vi "Calcu_STD Pressure_PC.vi"(6 "Resolution":string[][](array[string]), 7 "STD 단위":string, 8 "Cal STD (-)":string[](array[string]), 10 "Cal STD (+)":string[](array[string]), 11 "Condition":string[][](array[string])) -> (0 "배열":dbl[](array[numeric]), 3 "Data Out":string[][](array[string]), 5 "STD Data":string[][](array[string]))   [LabVIEW 2020]
uses:
  Variables/Global_Cal Info.vi
  <vilib>/express/express arith-compare/Formula/XNode/ExpressFormulaBlockNode.xnode
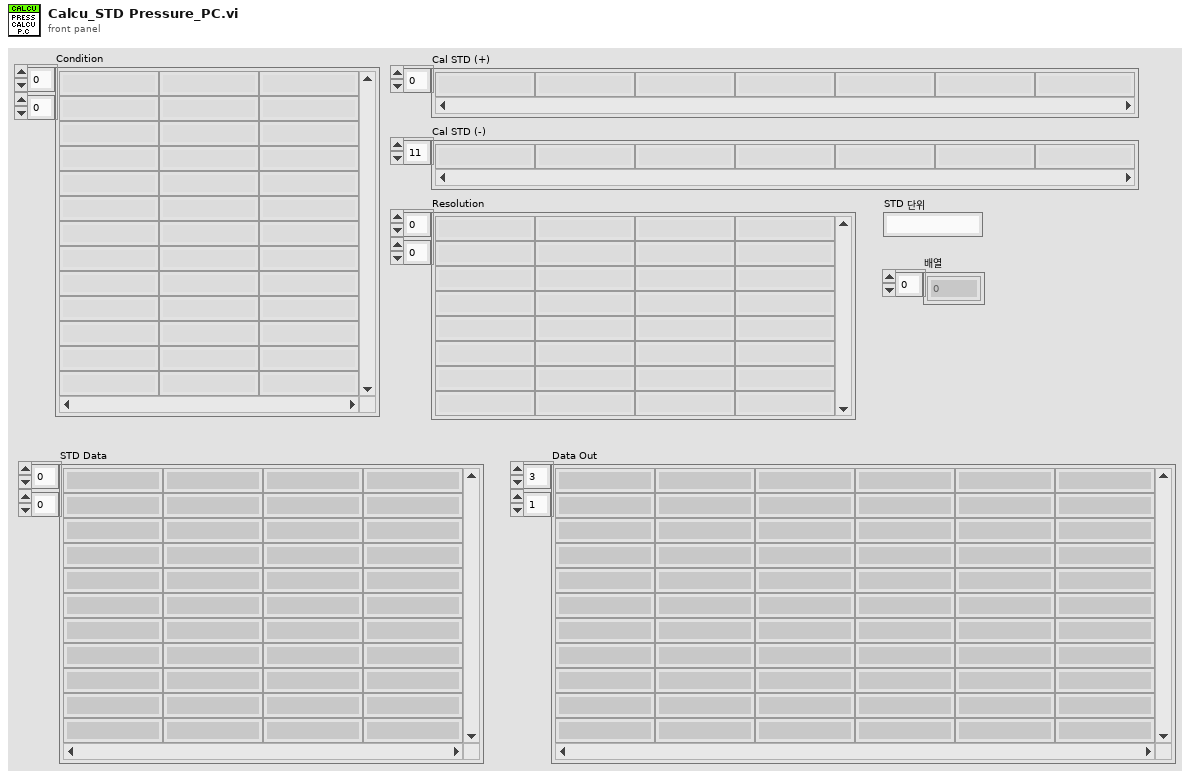
[diagram p1: front panel]
types:
  T1 = cluster{"세부분류코드":string, "형식":string, "옵션":string, "측정기명":string, "EXCEL파일명":string, "TEMP":string}
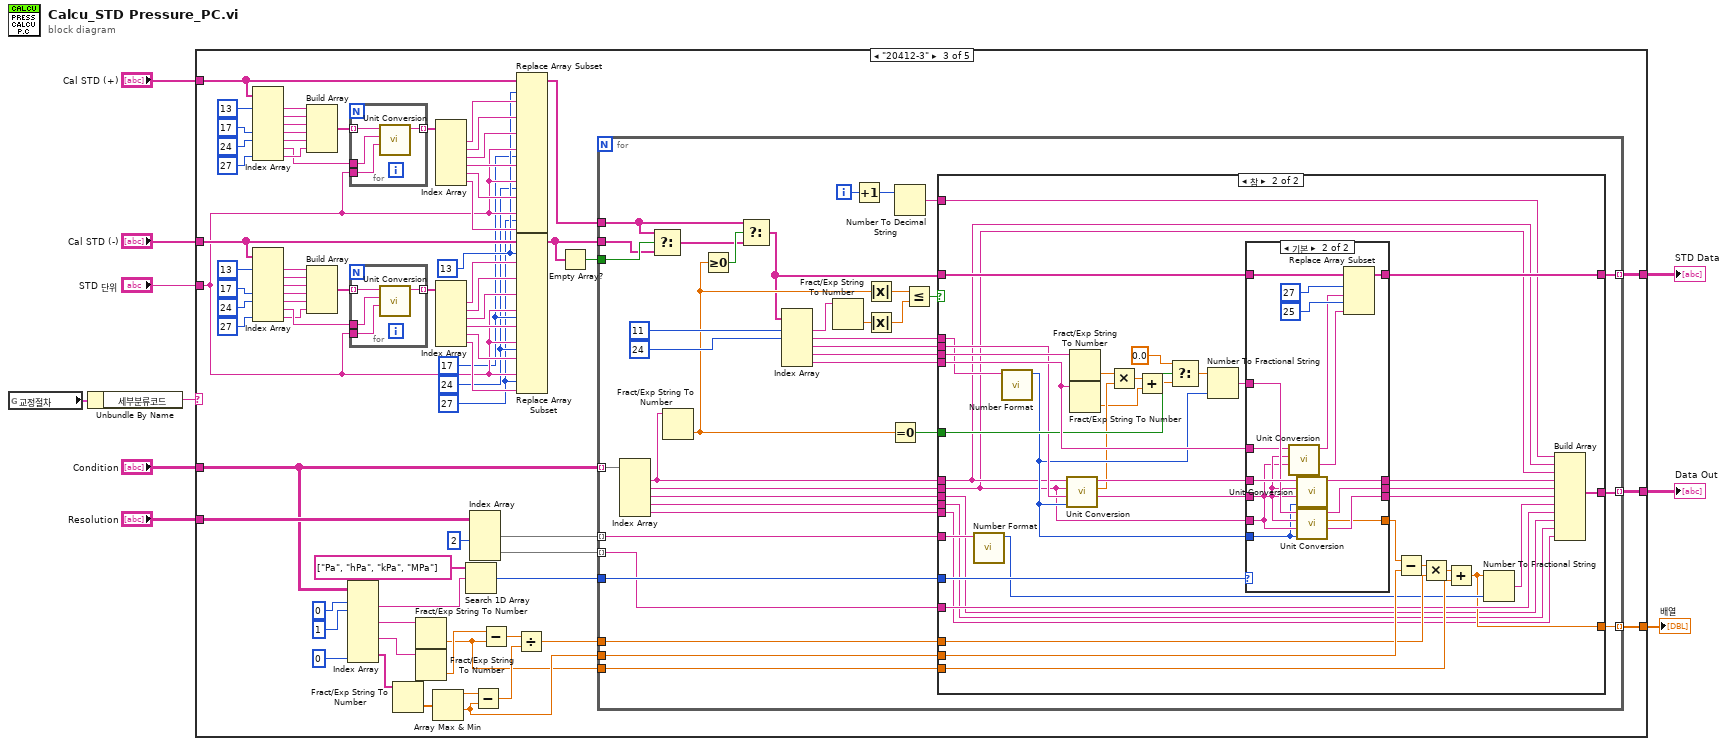
[diagram p0: block diagram]
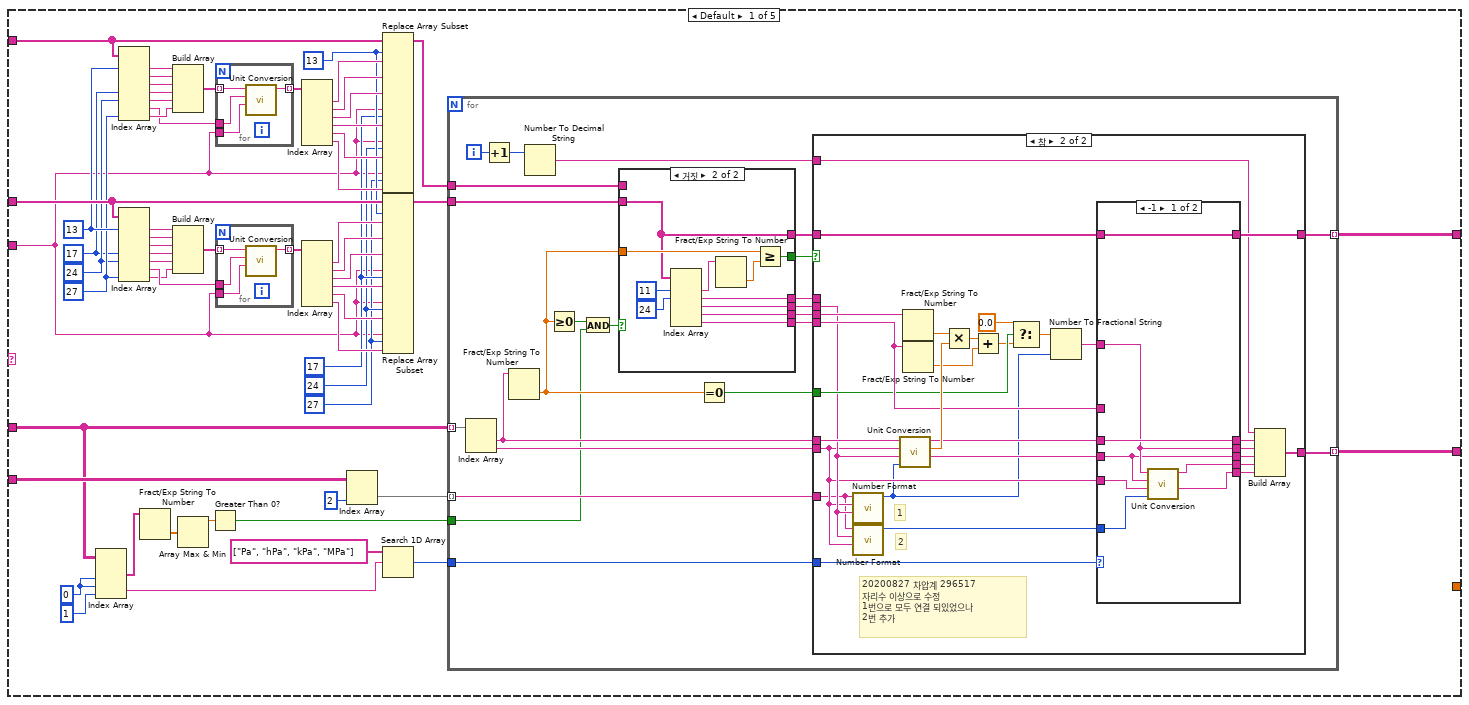
[diagram p2: hidden frame]
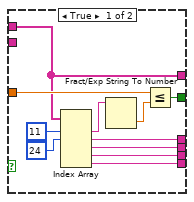
[diagram p3: hidden frame]
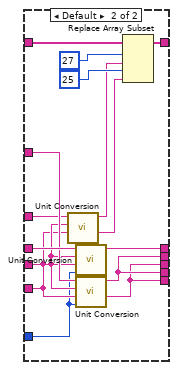
[diagram p5: hidden frame]
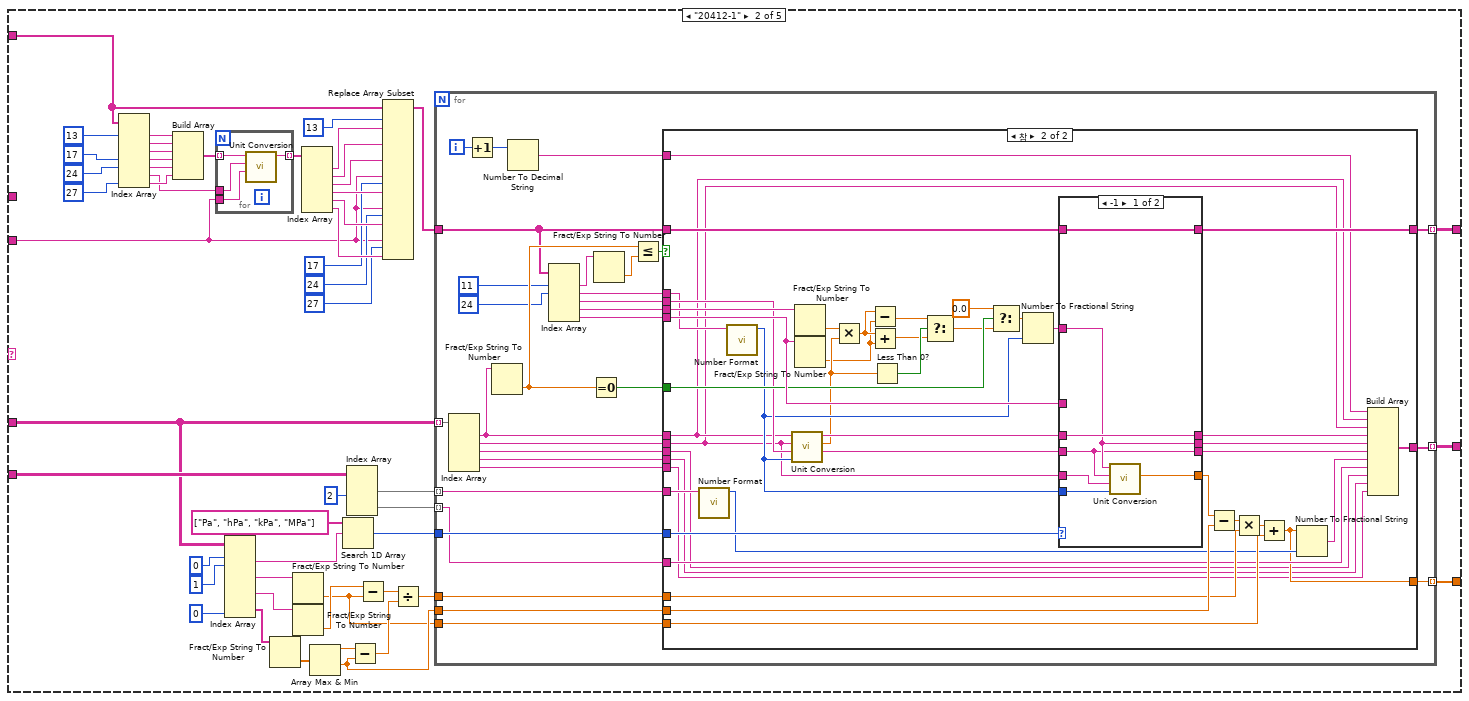
[diagram p6: hidden frame]
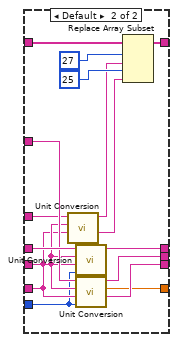
[diagram p8: hidden frame]
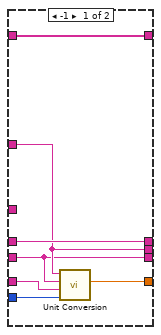
[diagram p10: hidden frame]
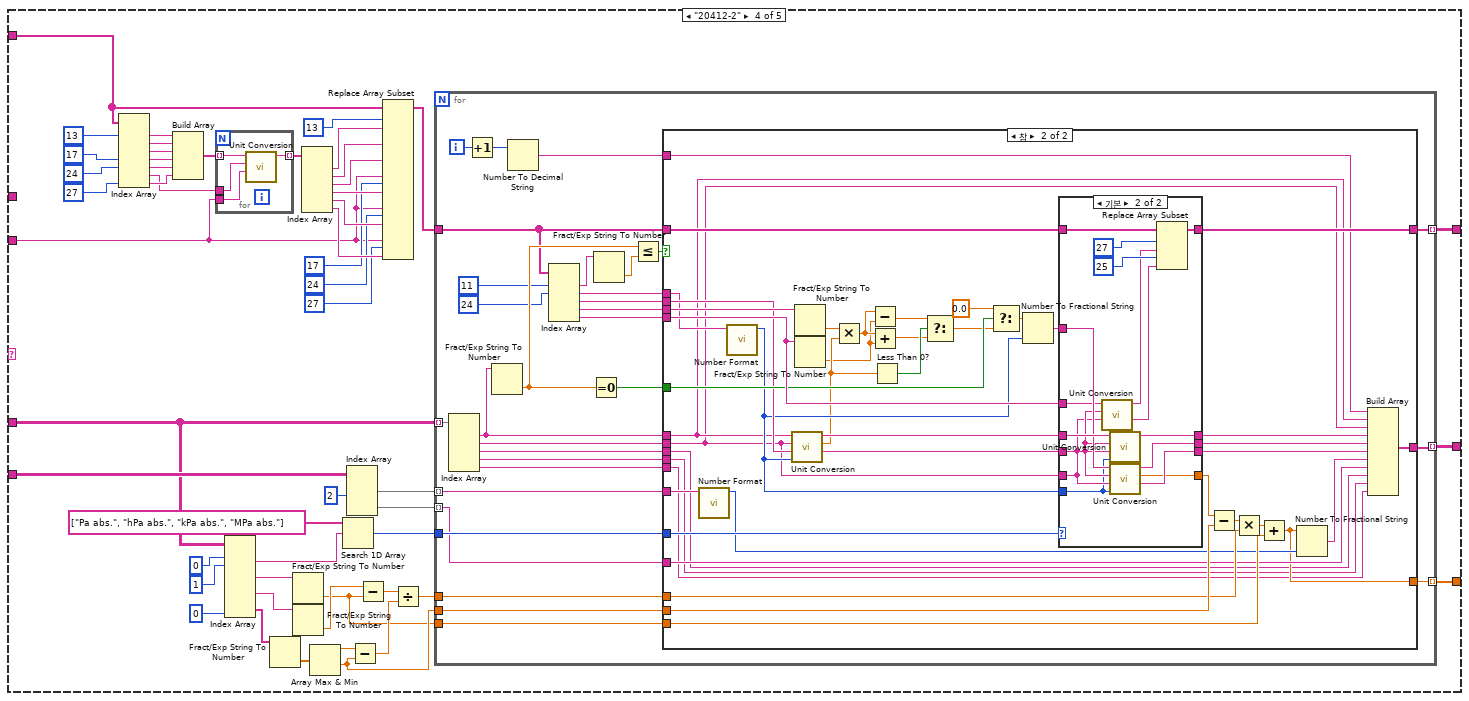
[diagram p11: hidden frame]
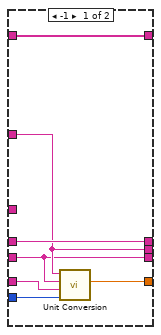
[diagram p13: hidden frame]
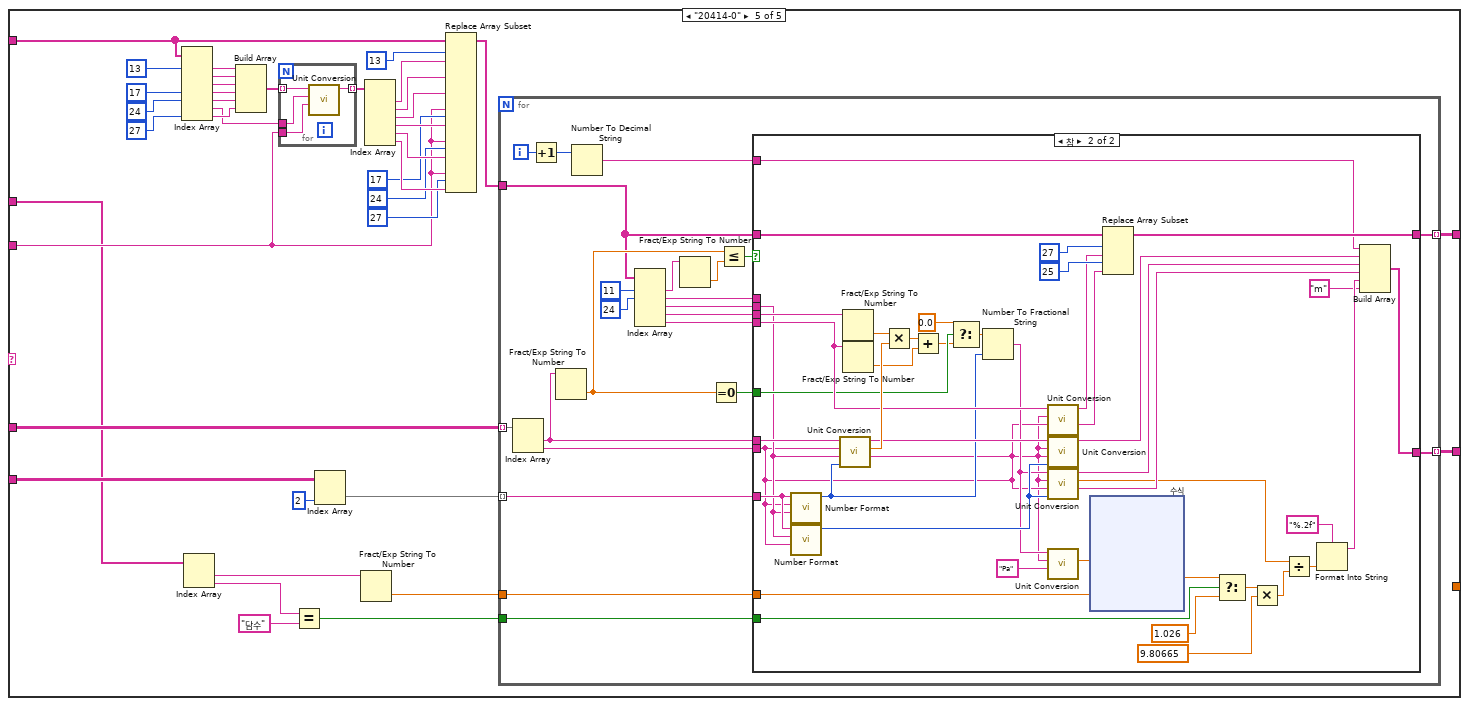
[diagram p14: hidden frame]
diagram:
  n1 = global read "Global_Cal Info.vi" "교정절차"() -> (w3:T1)
  n2 = Unbundle By Name(w3) -> ("세부분류코드"=w2:string)
  n3 = case shown="\"20412-3\"" w2 {
    tunnel: "Resolution" -> [w68 w224 w397 w556 w694]
    tunnel: [w61 w217 w390 w549 w691] -> w9
    tunnel: [w60 w216 w389 w548 w690] -> w8
    tunnel: "Condition" -> [w59 w215 w388 w547 w689]
    tunnel: "Cal STD (+)" -> [w43 w199 w372 w531 w665]
    tunnel: "Cal STD (-)" -> [w26 _ w332 _ w662]
    tunnel: "STD 단위" -> [w16 w189 w331 w521 w664]
    tunnel: [_ w174 w352 w506 _] -> w1
    frame Default {
      w23 = 17 ("인덱스")
      w21 = 27 ("인덱스")
      w22 = 24 ("인덱스")
      w24 = 13 ("인덱스")
      w17 = 17 ("인덱스")
      w19 = 27 ("인덱스")
      w18 = 24 ("인덱스")
      w20 = 13 ("인덱스")
      w11 = 0 ("비활성화된 인덱스 (열)")
      n4 = Index Array(array=w59, index (col) #1=w11, index (row) #2=w11, index (col) #2=1 ("인덱스 (행)")) -> (element #1=w13:string[], element #2=w66:string)  [unwired: 1 in]
      n5 = Index Array(array=w43, index #1=w20, index #4=w17, index #5=w18, index #7=w19) -> (element #1=w58:string, element #2=w57:string, element #3=w56:string, element #4=w54:string, element #5=w53:string, element #6=w52:string, element #7=w55:string)  [unwired: 3 in]
      n6 = Index Array(array=w26, index #1=w20, index #4=w17, index #5=w18, index #7=w19) -> (element #1=w27:string, element #2=w28:string, element #3=w29:string, element #4=w31:string, element #5=w32:string, element #6=w33:string, element #7=w30:string)  [unwired: 3 in]
      n7 = Fract/Exp String To Number(string=w13) -> (number=w14:dbl[])  [unwired: 3 in, 1 out]
      n8 = Build Array(w58, w57, w56, w54, w53, w55) -> (w51:string[])
      n9 = Build Array(w27, w28, w29, w31, w32, w30) -> (w34:string[])
      n10 = Array Max & Min(array=w14) -> (max value=w15:dbl)  [unwired: 3 out]
      n11 = Greater Than 0?(x=w15) -> (x > 0?=w12:bool)
      n12 = for {
        tunnel: w52 -> [w76]
        tunnel: w51 -> [w75] mode=indexing
        tunnel: w16 -> [w74]
        tunnel: [w73] -> w50 mode=indexing
        n13 = call "Unit Conversion.vi"("환산단위"=w74, "입력단위"=w76, "입력값"=w75) -> ("환산값 (string)"=w73:string)  [unwired: 3 in, 5 out]
      }
      n14 = for {
        tunnel: w33 -> [w72]
        tunnel: w34 -> [w71] mode=indexing
        tunnel: w16 -> [w70]
        tunnel: [w69] -> w35 mode=indexing
        n15 = call "Unit Conversion.vi"("환산단위"=w70, "입력단위"=w72, "입력값"=w71) -> ("환산값 (string)"=w69:string)  [unwired: 3 in, 5 out]
      }
      n16 = Index Array(array=w50) -> (element #1=w49:string, element #2=w48:string, element #3=w47:string, element #4=w46:string, element #5=w45:string, element #6=w44:string)  [unwired: 6 in]
      n17 = Index Array(array=w35) -> (element #1=w36:string, element #2=w37:string, element #3=w38:string, element #4=w39:string, element #5=w40:string, element #6=w41:string)  [unwired: 6 in]
      n18 = Index Array(array=w68, index (col)=2 ("비활성화된 인덱스 (열)")) -> (element=w62:string[])  [unwired: 1 in]
      n19 = Replace Array Subset(array=w43, new element #1=w49, index #1=w24, new element #2=w48, new element #3=w47, new element #4=w16, new element #5=w46, index #5=w23, new element #6=w16, new element #7=w45, index #7=w22, new element #8=w16, new element #9=w44, index #9=w21) -> (w42:string[])  [unwired: 5 in]
      n20 = Replace Array Subset(array=w26, new element #1=w36, index #1=w24, new element #2=w37, new element #3=w38, new element #4=w16, new element #5=w39, index #5=w23, new element #6=w16, new element #7=w40, index #7=w22, new element #8=w16, new element #9=w41, index #9=w21) -> (w25:string[])  [unwired: 5 in]
      n21 = Search 1D Array(1D array=string[] ["Pa", "hPa", "kPa", "MPa"], element=w66) -> (index of element=w67:i32)  [unwired: 1 in]
      n22 = for {
        tunnel: w59 -> [w99] mode=indexing
        tunnel: [w97] -> w60 mode=indexing
        tunnel: w42 -> [w98]
        tunnel: [w96] -> w61 mode=indexing
        tunnel: w62 -> [w92] mode=indexing
        tunnel: w67 -> [w93]
        tunnel: w25 -> [w88]
        tunnel: w12 -> [w77]
        i -> [w91]
        n23 = Index Array(array=w99) -> (element #1=w94:string, element #2=w95:string)  [unwired: 2 in]
        n24 = Increment(x=w91) -> (x+1=w90:i32)
        n25 = Fract/Exp String To Number(string=w94) -> (number=w87:dbl)  [unwired: 3 in, 1 out]
        n26 = Number To Decimal String(number=w90) -> (decimal integer string=w89:string)  [unwired: 1 in]
        n27 = Greater Or Equal To 0?(x=w87) -> (x >= 0?=w79:bool)
        n28 = And(x=w79, y=w77) -> (x .and. y?=w78:bool)
        n29 = case shown="거짓" w78 {
          tunnel: w98 -> [w100 _]
          tunnel: [w110 w121] -> w86
          tunnel: [w109 w120] -> w85
          tunnel: [w108 w119] -> w84
          tunnel: [w107 w118] -> w83
          tunnel: w87 -> [w106 w117]
          tunnel: [w101 w112] -> w82
          tunnel: w88 -> [_ w111]
          tunnel: [w100 w111] -> w81
          frame True {
            n30 = Index Array(array=w100, index #1=11 ("인덱스"), index #2=24 ("인덱스")) -> (element #1=w103:string, element #2=w101:string, element #3=w108:string, element #4=w107:string, element #5=w109:string)  [unwired: 3 in]
            n31 = Fract/Exp String To Number(string=w103) -> (number=w105:dbl)  [unwired: 3 in, 1 out]
            n32 = Less Or Equal?(x=w106, y=w105) -> (x <= y?=w110:bool)
          }
          frame False {
            n33 = Index Array(array=w111, index #1=11 ("인덱스"), index #2=24 ("인덱스")) -> (element #1=w114:string, element #2=w112:string, element #3=w119:string, element #4=w118:string, element #5=w120:string)  [unwired: 3 in]
            n34 = Fract/Exp String To Number(string=w114) -> (number=w116:dbl)  [unwired: 3 in, 1 out]
            n35 = Greater Or Equal?(x=w117, y=w116) -> (x >= y?=w121:bool)
          }
        }
        n36 = Equal To 0?(x=w87) -> (x = 0?=w80:bool)
        n37 = case shown="참" w86 {
          tunnel: [_ w149] -> w96
          tunnel: w89 -> [_ w134]
          tunnel: w81 -> [_ w137]
          tunnel: [_ w136] -> w97
          tunnel: w84 -> [_ w127]
          tunnel: w85 -> [_ w135]
          tunnel: w95 -> [_ w126]
          tunnel: w94 -> [_ w144]
          tunnel: w83 -> [_ w147]
          tunnel: w82 -> [_ _]
          tunnel: w93 -> [_ w143]
          tunnel: w92 -> [_ w122]
          tunnel: w80 -> [_ w133]
          frame False {
          }
          frame True {
            # "2"
            # "1"
            # "20200827 차압계 296517\n자리수 이상으로 수정\n1번으로 모두 연결 되있었으나\n2번 추가"
            n38 = call "Number Format.vi"("기준단위"=w127, "입력단위"=w126, "입력값"=w122) -> ("정밀도(단위적용)"=w123:i32)  [unwired: 8 in]
            n39 = call "Number Format.vi"("기준단위"=w126, "입력단위"=w127, "입력값"=w122) -> ("정밀도(단위적용)"=w124:i32)  [unwired: 8 in]
            n40 = call "Unit Conversion.vi"("소수점 자리수"=w123, "환산단위"=w127, "입력단위"=w126, "입력값"=w144) -> ("환산단위"=w128:string, "환산값 (DBL)"=w148:dbl, "환산값 (string)"=w129:string)  [unwired: 2 in, 3 out]
            n41 = Fract/Exp String To Number(string=w147) -> (number=w146:dbl)  [unwired: 3 in, 1 out]
            n42 = Fract/Exp String To Number(string=w135) -> (number=w145:dbl)  [unwired: 3 in, 1 out]
            n43 = Multiply(x=w146, y=w148) -> (x*y=w150:dbl)
            n44 = Add(x=w150, y=w145) -> (x+y=w132:dbl)
            n45 = Select(t=0.0, s=w133, f=w132) -> (s? t:f=w130:dbl)
            n46 = Number To Fractional String(number=w130, precision (6)=w123) -> (F-format string=w125:string)  [unwired: 2 in]
            n47 = case shown="-1" w143 {
              tunnel: w129 -> [w158 w173]
              tunnel: w126 -> [w151 w160]
              tunnel: w125 -> [w155 w172]
              tunnel: [w158 w171] -> w142
              tunnel: [w155 w170] -> w141
              tunnel: [w152 w169] -> w140
              tunnel: [w157 w170] -> w139
              tunnel: [w156 w169] -> w138
              tunnel: w124 -> [w154 w159]
              tunnel: w128 -> [w152 w161]
              tunnel: w137 -> [w153 w168]
              tunnel: [w153 w167] -> w136
              tunnel: w135 -> [_ w166]
              frame -1 {
                n48 = call "Unit Conversion.vi"("소수점 자리수"=w154, "환산단위"=w151, "입력단위"=w152, "입력값"=w155) -> ("환산단위"=w156:string, "환산값 (string)"=w157:string)  [unwired: 2 in, 4 out]
              }
              frame Default {
                n49 = call "Unit Conversion.vi"("환산단위"=w160, "입력단위"=w161, "입력값"=w166) -> ("환산단위"=w162:string, "환산값 (string)"=w163:string)  [unwired: 3 in, 4 out]
                n50 = call "Unit Conversion.vi"("소수점 자리수"=w159, "환산단위"=w160, "입력단위"=w161, "입력값"=w173) -> ("환산값 (string)"=w171:string)  [unwired: 2 in, 5 out]
                n51 = call "Unit Conversion.vi"("소수점 자리수"=w159, "환산단위"=w160, "입력단위"=w161, "입력값"=w172) -> ("환산단위"=w169:string, "환산값 (string)"=w170:string)  [unwired: 2 in, 4 out]
                n52 = Replace Array Subset(array=w168, new element #1=w163, index #1=27 ("인덱스"), new element #2=w162, index #2=25 ("인덱스")) -> (w167:string[])
              }
            }
            n53 = Build Array(w134, w142, w141, w140, w139, w138) -> (w149:string[])
          }
        }
      }
    }
    frame "20412-1" {
      n54 = Index Array(array=w199, index #1=13 ("인덱스"), index #4=17 ("인덱스"), index #5=24 ("인덱스"), index #7=27 ("인덱스")) -> (element #1=w214:string, element #2=w213:string, element #3=w212:string, element #4=w210:string, element #5=w209:string, element #6=w208:string, element #7=w211:string)  [unwired: 3 in]
      n55 = Build Array(w214, w213, w212, w210, w209, w211) -> (w207:string[])
      n56 = for {
        tunnel: w208 -> [w228]
        tunnel: w207 -> [w227] mode=indexing
        tunnel: w189 -> [w226]
        tunnel: [w225] -> w206 mode=indexing
        n57 = call "Unit Conversion.vi"("환산단위"=w226, "입력단위"=w228, "입력값"=w227) -> ("환산값 (string)"=w225:string)  [unwired: 3 in, 5 out]
      }
      n58 = Index Array(array=w215, index (row) #1=0 ("비활성화된 인덱스 (열)"), index (col) #1=1 ("인덱스 (행)"), index (col) #4=0 ("인덱스 (열)")) -> (element #1=w222:string, element #2=w187:string, element #3=w186:string, element #4=w183:string[])  [unwired: 5 in]
      n59 = Fract/Exp String To Number(string=w183) -> (number=w182:dbl[])  [unwired: 3 in, 1 out]
      n60 = Fract/Exp String To Number(string=w187) -> (number=w176:dbl)  [unwired: 3 in, 1 out]
      n61 = Fract/Exp String To Number(string=w186) -> (number=w185:dbl)  [unwired: 3 in, 1 out]
      n62 = Index Array(array=w206) -> (element #1=w205:string, element #2=w204:string, element #3=w203:string, element #4=w202:string, element #5=w201:string, element #6=w200:string)  [unwired: 6 in]
      n63 = Array Max & Min(array=w182) -> (max value=w181:dbl, min value=w177:dbl)  [unwired: 2 out]
      n64 = Search 1D Array(1D array=string[] ["Pa", "hPa", "kPa", "MPa"], element=w222) -> (index of element=w223:i32)  [unwired: 1 in]
      n65 = Index Array(array=w224, index (col) #1=2 ("비활성화된 인덱스 (열)")) -> (element #1=w218:string[], element #2=w175:string[])  [unwired: 3 in]
      n66 = Subtract(x=w181, y=w177) -> (x-y=w179:dbl)
      n67 = Subtract(x=w185, y=w176) -> (x-y=w180:dbl)
      n68 = Replace Array Subset(array=w199, new element #1=w205, index #1=13 ("인덱스"), new element #2=w204, new element #3=w203, new element #4=w189, new element #5=w202, index #5=17 ("인덱스"), new element #6=w189, new element #7=w201, index #7=24 ("인덱스"), new element #8=w189, new element #9=w200, index #9=27 ("인덱스")) -> (w198:string[])  [unwired: 5 in]
      n69 = Divide(x=w180, y=w179) -> (x/y=w178:dbl)
      n70 = for {
        tunnel: w215 -> [w258] mode=indexing
        tunnel: [w257] -> w216 mode=indexing
        tunnel: w198 -> [w242]
        tunnel: [w256] -> w217 mode=indexing
        tunnel: w218 -> [w252] mode=indexing
        tunnel: w223 -> [w253]
        tunnel: w178 -> [w240]
        tunnel: w177 -> [w239]
        tunnel: w176 -> [w238]
        tunnel: w175 -> [w237] mode=indexing
        tunnel: [w236] -> w174 mode=indexing
        i -> [w251]
        n71 = Index Array(array=w258) -> (element #1=w254:string, element #2=w255:string, element #3=w235:string, element #4=w234:string, element #5=w233:string)  [unwired: 5 in]
        n72 = Increment(x=w251) -> (x+1=w250:i32)
        n73 = Fract/Exp String To Number(string=w254) -> (number=w248:dbl)  [unwired: 3 in, 1 out]
        n74 = Number To Decimal String(number=w250) -> (decimal integer string=w249:string)  [unwired: 1 in]
        n75 = Index Array(array=w242, index #1=11 ("인덱스"), index #2=24 ("인덱스")) -> (element #1=w230:string, element #2=w243:string, element #3=w245:string, element #4=w244:string, element #5=w246:string)  [unwired: 3 in]
        n76 = Equal To 0?(x=w248) -> (x = 0?=w241:bool)
        n77 = Fract/Exp String To Number(string=w230) -> (number=w232:dbl)  [unwired: 3 in, 1 out]
        n78 = Less Or Equal?(x=w248, y=w232) -> (x <= y?=w247:bool)
        n79 = case shown="참" w247 {
          tunnel: [_ w301] -> w256
          tunnel: w249 -> [_ w288]
          tunnel: w242 -> [_ w292]
          tunnel: [_ w291] -> w257
          tunnel: w245 -> [_ w284]
          tunnel: w246 -> [_ w290]
          tunnel: w255 -> [_ w259]
          tunnel: w254 -> [_ w260]
          tunnel: w244 -> [_ w300]
          tunnel: w243 -> [_ w274]
          tunnel: w253 -> [_ w298]
          tunnel: w252 -> [_ w273]
          tunnel: w241 -> [_ w287]
          tunnel: w240 -> [_ w280]
          tunnel: w239 -> [_ w282]
          tunnel: w238 -> [_ w278]
          tunnel: w237 -> [_ w275]
          tunnel: [_ w271] -> w236
          tunnel: w235 -> [_ w270]
          tunnel: w234 -> [_ w269]
          tunnel: w233 -> [_ w268]
          frame False {
          }
          frame True {
            n80 = call "Number Format.vi"("입력값"=w273) -> ("정밀도(단위적용)"=w272:i32)  [unwired: 10 in]
            n81 = call "Number Format.vi"("입력값"=w274) -> ("정밀도(단위적용)"=w276:i32)  [unwired: 10 in]
            n82 = call "Unit Conversion.vi"("소수점 자리수"=w276, "환산단위"=w284, "입력단위"=w259, "입력값"=w260) -> ("환산단위"=w289:string, "환산값 (DBL)"=w267:dbl, "환산값 (string)"=w297:string)  [unwired: 2 in, 3 out]
            n83 = Fract/Exp String To Number(string=w300) -> (number=w299:dbl)  [unwired: 3 in, 1 out]
            n84 = Fract/Exp String To Number(string=w290) -> (number=w265:dbl)  [unwired: 3 in, 1 out]
            n85 = Multiply(x=w299, y=w267) -> (x*y=w266:dbl)
            n86 = Subtract(x=w266, y=w265) -> (x-y=w262:dbl)
            n87 = Add(x=w266, y=w265) -> (x+y=w261:dbl)
            n88 = Less Than 0?(x=w267) -> (x < 0?=w264:bool)
            n89 = Select(t=w262, s=w264, f=w261) -> (s? t:f=w263:dbl)
            n90 = Select(t=0.0, s=w287, f=w263) -> (s? t:f=w285:dbl)
            n91 = Number To Fractional String(number=w285, precision (6)=w276) -> (F-format string=w296:string)  [unwired: 2 in]
            n92 = case shown="-1" w298 {
              tunnel: w297 -> [w308 w324]
              tunnel: w259 -> [w304 w311]
              tunnel: w296 -> [w307 w323]
              tunnel: [w308 w322] -> w295
              tunnel: [w307 w321] -> w294
              tunnel: [w305 w320] -> w293
              tunnel: w276 -> [w302 w310]
              tunnel: w289 -> [w305 w312]
              tunnel: w292 -> [w306 w319]
              tunnel: [w306 w318] -> w291
              tunnel: w290 -> [_ w317]
              tunnel: [w303 w309] -> w283
              frame -1 {
                n93 = call "Unit Conversion.vi"("소수점 자리수"=w302, "환산단위"=w304, "입력단위"=w305, "입력값"=w307) -> ("환산값 (DBL)"=w303:dbl)  [unwired: 2 in, 5 out]
              }
              frame Default {
                n94 = call "Unit Conversion.vi"("환산단위"=w311, "입력단위"=w312, "입력값"=w317) -> ("환산단위"=w313:string, "환산값 (string)"=w314:string)  [unwired: 3 in, 4 out]
                n95 = call "Unit Conversion.vi"("소수점 자리수"=w310, "환산단위"=w311, "입력단위"=w312, "입력값"=w324) -> ("환산값 (string)"=w322:string)  [unwired: 2 in, 5 out]
                n96 = call "Unit Conversion.vi"("소수점 자리수"=w310, "환산단위"=w311, "입력단위"=w312, "입력값"=w323) -> ("환산단위"=w320:string, "환산값 (DBL)"=w309:dbl, "환산값 (string)"=w321:string)  [unwired: 2 in, 3 out]
                n97 = Replace Array Subset(array=w319, new element #1=w314, index #1=27 ("인덱스"), new element #2=w313, index #2=25 ("인덱스")) -> (w318:string[])
              }
            }
            n98 = Subtract(x=w283, y=w282) -> (x-y=w281:dbl)
            n99 = Multiply(x=w281, y=w280) -> (x*y=w279:dbl)
            n100 = Add(x=w279, y=w278) -> (x+y=w271:dbl)
            n101 = Number To Fractional String(number=w271, precision (6)=w272) -> (F-format string=w277:string)  [unwired: 2 in]
            n102 = Build Array(w288, w260, w259, w295, w294, w293, w277, w275, w270, w269, w268) -> (w301:string[])
          }
        }
      }
    }
    frame "20412-3" {
      w329 = 17 ("인덱스")
      w327 = 27 ("인덱스")
      w328 = 24 ("인덱스")
      w330 = 13 ("인덱스")
      n103 = Index Array(array=w372, index #1=13 ("인덱스"), index #4=17 ("인덱스"), index #5=24 ("인덱스"), index #7=27 ("인덱스")) -> (element #1=w387:string, element #2=w386:string, element #3=w385:string, element #4=w383:string, element #5=w382:string, element #6=w381:string, element #7=w384:string)  [unwired: 3 in]
      n104 = Index Array(array=w332, index #1=13 ("인덱스"), index #4=17 ("인덱스"), index #5=24 ("인덱스"), index #7=27 ("인덱스")) -> (element #1=w333:string, element #2=w334:string, element #3=w335:string, element #4=w337:string, element #5=w338:string, element #6=w339:string, element #7=w336:string)  [unwired: 3 in]
      n105 = Build Array(w387, w386, w385, w383, w382, w384) -> (w380:string[])
      n106 = Build Array(w333, w334, w335, w337, w338, w336) -> (w340:string[])
      n107 = Index Array(array=w388, index (row) #1=0 ("비활성화된 인덱스 (열)"), index (col) #1=1 ("인덱스 (행)"), index (col) #4=0 ("인덱스 (열)")) -> (element #1=w395:string, element #2=w365:string, element #3=w364:string, element #4=w361:string[])  [unwired: 5 in]
      n108 = for {
        tunnel: w381 -> [w405]
        tunnel: w380 -> [w404] mode=indexing
        tunnel: w331 -> [w403]
        tunnel: [w402] -> w379 mode=indexing
        n109 = call "Unit Conversion.vi"("환산단위"=w403, "입력단위"=w405, "입력값"=w404) -> ("환산값 (string)"=w402:string)  [unwired: 3 in, 5 out]
      }
      n110 = for {
        tunnel: w339 -> [w401]
        tunnel: w340 -> [w400] mode=indexing
        tunnel: w331 -> [w399]
        tunnel: [w398] -> w341 mode=indexing
        n111 = call "Unit Conversion.vi"("환산단위"=w399, "입력단위"=w401, "입력값"=w400) -> ("환산값 (string)"=w398:string)  [unwired: 3 in, 5 out]
      }
      n112 = Fract/Exp String To Number(string=w361) -> (number=w360:dbl[])  [unwired: 3 in, 1 out]
      n113 = Fract/Exp String To Number(string=w365) -> (number=w354:dbl)  [unwired: 3 in, 1 out]
      n114 = Fract/Exp String To Number(string=w364) -> (number=w363:dbl)  [unwired: 3 in, 1 out]
      n115 = Array Max & Min(array=w360) -> (max value=w359:dbl, min value=w355:dbl)  [unwired: 2 out]
      n116 = Index Array(array=w379) -> (element #1=w378:string, element #2=w377:string, element #3=w376:string, element #4=w375:string, element #5=w374:string, element #6=w373:string)  [unwired: 6 in]
      n117 = Index Array(array=w341) -> (element #1=w342:string, element #2=w343:string, element #3=w344:string, element #4=w345:string, element #5=w346:string, element #6=w347:string)  [unwired: 6 in]
      n118 = Search 1D Array(1D array=string[] ["Pa", "hPa", "kPa", "MPa"], element=w395) -> (index of element=w396:i32)  [unwired: 1 in]
      n119 = Index Array(array=w397, index (col) #1=2 ("비활성화된 인덱스 (열)")) -> (element #1=w391:string[], element #2=w353:string[])  [unwired: 3 in]
      n120 = Subtract(x=w359, y=w355) -> (x-y=w357:dbl)
      n121 = Subtract(x=w363, y=w354) -> (x-y=w358:dbl)
      n122 = Divide(x=w358, y=w357) -> (x/y=w356:dbl)
      n123 = Replace Array Subset(array=w372, new element #1=w378, index #1=w330, new element #2=w377, new element #3=w376, new element #4=w331, new element #5=w375, index #5=w329, new element #6=w331, new element #7=w374, index #7=w328, new element #8=w331, new element #9=w373, index #9=w327) -> (w371:string[])  [unwired: 5 in]
      n124 = Replace Array Subset(array=w332, new element #1=w342, index #1=w330, new element #2=w343, new element #3=w344, new element #4=w331, new element #5=w345, index #5=w329, new element #6=w331, new element #7=w346, index #7=w328, new element #8=w331, new element #9=w347, index #9=w327) -> (w326:string[])  [unwired: 5 in]
      n125 = Empty Array?(array=w326) -> (empty?=w325:bool)
      n126 = for {
        tunnel: w388 -> [w442] mode=indexing
        tunnel: [w441] -> w389 mode=indexing
        tunnel: w371 -> [w410]
        tunnel: [w440] -> w390 mode=indexing
        tunnel: w391 -> [w436] mode=indexing
        tunnel: w396 -> [w437]
        tunnel: w356 -> [w426]
        tunnel: w355 -> [w425]
        tunnel: w354 -> [w424]
        tunnel: w353 -> [w423] mode=indexing
        tunnel: [w422] -> w352 mode=indexing
        tunnel: w326 -> [w409]
        tunnel: w325 -> [w411]
        i -> [w435]
        n127 = Index Array(array=w442) -> (element #1=w438:string, element #2=w439:string, element #3=w421:string, element #4=w420:string, element #5=w419:string)  [unwired: 5 in]
        n128 = Select(t=w410, s=w411, f=w409) -> (s? t:f=w408:string[])
        n129 = Fract/Exp String To Number(string=w438) -> (number=w414:dbl)  [unwired: 3 in, 1 out]
        n130 = Greater Or Equal To 0?(x=w414) -> (x >= 0?=w413:bool)
        n131 = Select(t=w410, s=w413, f=w408) -> (s? t:f=w412:string[])
        n132 = Index Array(array=w412, index #1=11 ("인덱스"), index #2=24 ("인덱스")) -> (element #1=w416:string, element #2=w428:string, element #3=w430:string, element #4=w429:string, element #5=w431:string)  [unwired: 3 in]
        n133 = Fract/Exp String To Number(string=w416) -> (number=w418:dbl)  [unwired: 3 in, 1 out]
        n134 = Increment(x=w435) -> (x+1=w434:i32)
        n135 = Absolute Value(x=w414) -> (abs(x)=w406:dbl)
        n136 = Absolute Value(x=w418) -> (abs(x)=w407:dbl)
        n137 = Equal To 0?(x=w414) -> (x = 0?=w427:bool)
        n138 = Number To Decimal String(number=w434) -> (decimal integer string=w433:string)  [unwired: 1 in]
        n139 = Less Or Equal?(x=w406, y=w407) -> (x <= y?=w432:bool)
        n140 = case shown="참" w432 {
          tunnel: [_ w482] -> w440
          tunnel: w433 -> [_ w469]
          tunnel: w412 -> [_ w473]
          tunnel: [_ w472] -> w441
          tunnel: w430 -> [_ w465]
          tunnel: w431 -> [_ w471]
          tunnel: w439 -> [_ w444]
          tunnel: w438 -> [_ w445]
          tunnel: w429 -> [_ w481]
          tunnel: w428 -> [_ w455]
          tunnel: w437 -> [_ w479]
          tunnel: w436 -> [_ w454]
          tunnel: w427 -> [_ w468]
          tunnel: w426 -> [_ w461]
          tunnel: w425 -> [_ w463]
          tunnel: w424 -> [_ w459]
          tunnel: w423 -> [_ w456]
          tunnel: [_ w452] -> w422
          tunnel: w421 -> [_ w451]
          tunnel: w420 -> [_ w450]
          tunnel: w419 -> [_ w449]
          frame False {
          }
          frame True {
            n141 = call "Number Format.vi"("입력값"=w454) -> ("정밀도(단위적용)"=w453:i32)  [unwired: 10 in]
            n142 = call "Number Format.vi"("입력값"=w455) -> ("정밀도(단위적용)"=w457:i32)  [unwired: 10 in]
            n143 = call "Unit Conversion.vi"("소수점 자리수"=w457, "환산단위"=w465, "입력단위"=w444, "입력값"=w445) -> ("환산단위"=w470:string, "환산값 (DBL)"=w448:dbl, "환산값 (string)"=w478:string)  [unwired: 2 in, 3 out]
            n144 = Fract/Exp String To Number(string=w481) -> (number=w480:dbl)  [unwired: 3 in, 1 out]
            n145 = Fract/Exp String To Number(string=w471) -> (number=w446:dbl)  [unwired: 3 in, 1 out]
            n146 = Multiply(x=w480, y=w448) -> (x*y=w447:dbl)
            n147 = Add(x=w447, y=w446) -> (x+y=w443:dbl)
            n148 = Select(t=0.0, s=w468, f=w443) -> (s? t:f=w466:dbl)
            n149 = Number To Fractional String(number=w466, precision (6)=w457) -> (F-format string=w477:string)  [unwired: 2 in]
            n150 = case shown="기본" w479 {
              tunnel: w478 -> [w489 w505]
              tunnel: w444 -> [w485 w492]
              tunnel: w477 -> [w488 w504]
              tunnel: [w489 w503] -> w476
              tunnel: [w488 w502] -> w475
              tunnel: [w486 w501] -> w474
              tunnel: w457 -> [w483 w491]
              tunnel: w470 -> [w486 w493]
              tunnel: w473 -> [w487 w500]
              tunnel: [w487 w499] -> w472
              tunnel: w471 -> [_ w498]
              tunnel: [w484 w490] -> w464
              frame -1 {
                n151 = call "Unit Conversion.vi"("소수점 자리수"=w483, "환산단위"=w485, "입력단위"=w486, "입력값"=w488) -> ("환산값 (DBL)"=w484:dbl)  [unwired: 2 in, 5 out]
              }
              frame Default {
                n152 = call "Unit Conversion.vi"("환산단위"=w492, "입력단위"=w493, "입력값"=w498) -> ("환산단위"=w494:string, "환산값 (string)"=w495:string)  [unwired: 3 in, 4 out]
                n153 = call "Unit Conversion.vi"("소수점 자리수"=w491, "환산단위"=w492, "입력단위"=w493, "입력값"=w505) -> ("환산값 (string)"=w503:string)  [unwired: 2 in, 5 out]
                n154 = call "Unit Conversion.vi"("소수점 자리수"=w491, "환산단위"=w492, "입력단위"=w493, "입력값"=w504) -> ("환산단위"=w501:string, "환산값 (DBL)"=w490:dbl, "환산값 (string)"=w502:string)  [unwired: 2 in, 3 out]
                n155 = Replace Array Subset(array=w500, new element #1=w495, index #1=27 ("인덱스"), new element #2=w494, index #2=25 ("인덱스")) -> (w499:string[])
              }
            }
            n156 = Subtract(x=w464, y=w463) -> (x-y=w462:dbl)
            n157 = Multiply(x=w462, y=w461) -> (x*y=w460:dbl)
            n158 = Add(x=w460, y=w459) -> (x+y=w452:dbl)
            n159 = Number To Fractional String(number=w452, precision (6)=w453) -> (F-format string=w458:string)  [unwired: 2 in]
            n160 = Build Array(w469, w445, w444, w476, w475, w474, w458, w456, w451, w450, w449) -> (w482:string[])
          }
        }
      }
    }
    frame "20412-2" {
      n161 = Index Array(array=w531, index #1=13 ("인덱스"), index #4=17 ("인덱스"), index #5=24 ("인덱스"), index #7=27 ("인덱스")) -> (element #1=w546:string, element #2=w545:string, element #3=w544:string, element #4=w542:string, element #5=w541:string, element #6=w540:string, element #7=w543:string)  [unwired: 3 in]
      n162 = Build Array(w546, w545, w544, w542, w541, w543) -> (w539:string[])
      n163 = for {
        tunnel: w540 -> [w560]
        tunnel: w539 -> [w559] mode=indexing
        tunnel: w521 -> [w558]
        tunnel: [w557] -> w538 mode=indexing
        n164 = call "Unit Conversion.vi"("환산단위"=w558, "입력단위"=w560, "입력값"=w559) -> ("환산값 (string)"=w557:string)  [unwired: 3 in, 5 out]
      }
      n165 = Index Array(array=w547, index (row) #1=0 ("비활성화된 인덱스 (열)"), index (col) #1=1 ("인덱스 (행)"), index (col) #4=0 ("인덱스 (열)")) -> (element #1=w554:string, element #2=w519:string, element #3=w518:string, element #4=w515:string[])  [unwired: 5 in]
      n166 = Fract/Exp String To Number(string=w515) -> (number=w514:dbl[])  [unwired: 3 in, 1 out]
      n167 = Fract/Exp String To Number(string=w519) -> (number=w508:dbl)  [unwired: 3 in, 1 out]
      n168 = Fract/Exp String To Number(string=w518) -> (number=w517:dbl)  [unwired: 3 in, 1 out]
      n169 = Index Array(array=w538) -> (element #1=w537:string, element #2=w536:string, element #3=w535:string, element #4=w534:string, element #5=w533:string, element #6=w532:string)  [unwired: 6 in]
      n170 = Array Max & Min(array=w514) -> (max value=w513:dbl, min value=w509:dbl)  [unwired: 2 out]
      n171 = Search 1D Array(1D array=string[] ["Pa abs.", "hPa abs.", "kPa abs.", "MPa abs."], element=w554) -> (index of element=w555:i32)  [unwired: 1 in]
      n172 = Index Array(array=w556, index (col) #1=2 ("비활성화된 인덱스 (열)")) -> (element #1=w550:string[], element #2=w507:string[])  [unwired: 3 in]
      n173 = Subtract(x=w513, y=w509) -> (x-y=w511:dbl)
      n174 = Subtract(x=w517, y=w508) -> (x-y=w512:dbl)
      n175 = Replace Array Subset(array=w531, new element #1=w537, index #1=13 ("인덱스"), new element #2=w536, new element #3=w535, new element #4=w521, new element #5=w534, index #5=17 ("인덱스"), new element #6=w521, new element #7=w533, index #7=24 ("인덱스"), new element #8=w521, new element #9=w532, index #9=27 ("인덱스")) -> (w530:string[])  [unwired: 5 in]
      n176 = Divide(x=w512, y=w511) -> (x/y=w510:dbl)
      n177 = for {
        tunnel: w547 -> [w590] mode=indexing
        tunnel: [w589] -> w548 mode=indexing
        tunnel: w530 -> [w574]
        tunnel: [w588] -> w549 mode=indexing
        tunnel: w550 -> [w584] mode=indexing
        tunnel: w555 -> [w585]
        tunnel: w510 -> [w572]
        tunnel: w509 -> [w571]
        tunnel: w508 -> [w570]
        tunnel: w507 -> [w569] mode=indexing
        tunnel: [w568] -> w506 mode=indexing
        i -> [w583]
        n178 = Index Array(array=w590) -> (element #1=w586:string, element #2=w587:string, element #3=w567:string, element #4=w566:string, element #5=w565:string)  [unwired: 5 in]
        n179 = Increment(x=w583) -> (x+1=w582:i32)
        n180 = Fract/Exp String To Number(string=w586) -> (number=w580:dbl)  [unwired: 3 in, 1 out]
        n181 = Number To Decimal String(number=w582) -> (decimal integer string=w581:string)  [unwired: 1 in]
        n182 = Index Array(array=w574, index #1=11 ("인덱스"), index #2=24 ("인덱스")) -> (element #1=w562:string, element #2=w575:string, element #3=w577:string, element #4=w576:string, element #5=w578:string)  [unwired: 3 in]
        n183 = Equal To 0?(x=w580) -> (x = 0?=w573:bool)
        n184 = Fract/Exp String To Number(string=w562) -> (number=w564:dbl)  [unwired: 3 in, 1 out]
        n185 = Less Or Equal?(x=w580, y=w564) -> (x <= y?=w579:bool)
        n186 = case shown="참" w579 {
          tunnel: [_ w633] -> w588
          tunnel: w581 -> [_ w620]
          tunnel: w574 -> [_ w624]
          tunnel: [_ w623] -> w589
          tunnel: w577 -> [_ w616]
          tunnel: w578 -> [_ w622]
          tunnel: w587 -> [_ w591]
          tunnel: w586 -> [_ w592]
          tunnel: w576 -> [_ w632]
          tunnel: w575 -> [_ w606]
          tunnel: w585 -> [_ w630]
          tunnel: w584 -> [_ w605]
          tunnel: w573 -> [_ w619]
          tunnel: w572 -> [_ w612]
          tunnel: w571 -> [_ w614]
          tunnel: w570 -> [_ w610]
          tunnel: w569 -> [_ w607]
          tunnel: [_ w603] -> w568
          tunnel: w567 -> [_ w602]
          tunnel: w566 -> [_ w601]
          tunnel: w565 -> [_ w600]
          frame False {
          }
          frame True {
            n187 = call "Number Format.vi"("입력값"=w605) -> ("정밀도(단위적용)"=w604:i32)  [unwired: 10 in]
            n188 = call "Number Format.vi"("입력값"=w606) -> ("정밀도(단위적용)"=w608:i32)  [unwired: 10 in]
            n189 = call "Unit Conversion.vi"("소수점 자리수"=w608, "환산단위"=w616, "입력단위"=w591, "입력값"=w592) -> ("환산단위"=w621:string, "환산값 (DBL)"=w599:dbl, "환산값 (string)"=w629:string)  [unwired: 2 in, 3 out]
            n190 = Fract/Exp String To Number(string=w632) -> (number=w631:dbl)  [unwired: 3 in, 1 out]
            n191 = Fract/Exp String To Number(string=w622) -> (number=w597:dbl)  [unwired: 3 in, 1 out]
            n192 = Multiply(x=w631, y=w599) -> (x*y=w598:dbl)
            n193 = Subtract(x=w598, y=w597) -> (x-y=w594:dbl)
            n194 = Add(x=w598, y=w597) -> (x+y=w593:dbl)
            n195 = Less Than 0?(x=w599) -> (x < 0?=w596:bool)
            n196 = Select(t=w594, s=w596, f=w593) -> (s? t:f=w595:dbl)
            n197 = Select(t=0.0, s=w619, f=w595) -> (s? t:f=w617:dbl)
            n198 = Number To Fractional String(number=w617, precision (6)=w608) -> (F-format string=w628:string)  [unwired: 2 in]
            n199 = case shown="기본" w630 {
              tunnel: w629 -> [w640 w656]
              tunnel: w591 -> [w636 w643]
              tunnel: w628 -> [w639 w655]
              tunnel: [w640 w654] -> w627
              tunnel: [w639 w653] -> w626
              tunnel: [w637 w652] -> w625
              tunnel: w608 -> [w634 w642]
              tunnel: w621 -> [w637 w644]
              tunnel: w624 -> [w638 w651]
              tunnel: [w638 w650] -> w623
              tunnel: w622 -> [_ w649]
              tunnel: [w635 w641] -> w615
              frame -1 {
                n200 = call "Unit Conversion.vi"("소수점 자리수"=w634, "환산단위"=w636, "입력단위"=w637, "입력값"=w639) -> ("환산값 (DBL)"=w635:dbl)  [unwired: 2 in, 5 out]
              }
              frame Default {
                n201 = call "Unit Conversion.vi"("환산단위"=w643, "입력단위"=w644, "입력값"=w649) -> ("환산단위"=w645:string, "환산값 (string)"=w646:string)  [unwired: 3 in, 4 out]
                n202 = call "Unit Conversion.vi"("소수점 자리수"=w642, "환산단위"=w643, "입력단위"=w644, "입력값"=w656) -> ("환산값 (string)"=w654:string)  [unwired: 2 in, 5 out]
                n203 = call "Unit Conversion.vi"("소수점 자리수"=w642, "환산단위"=w643, "입력단위"=w644, "입력값"=w655) -> ("환산단위"=w652:string, "환산값 (DBL)"=w641:dbl, "환산값 (string)"=w653:string)  [unwired: 2 in, 3 out]
                n204 = Replace Array Subset(array=w651, new element #1=w646, index #1=27 ("인덱스"), new element #2=w645, index #2=25 ("인덱스")) -> (w650:string[])
              }
            }
            n205 = Subtract(x=w615, y=w614) -> (x-y=w613:dbl)
            n206 = Multiply(x=w613, y=w612) -> (x*y=w611:dbl)
            n207 = Add(x=w611, y=w610) -> (x+y=w603:dbl)
            n208 = Number To Fractional String(number=w603, precision (6)=w604) -> (F-format string=w609:string)  [unwired: 2 in]
            n209 = Build Array(w620, w592, w591, w627, w626, w625, w609, w607, w602, w601, w600) -> (w633:string[])
          }
        }
      }
    }
    frame "20414-0" {
      n210 = Index Array(array=w665, index #1=13 ("인덱스"), index #4=17 ("인덱스"), index #5=24 ("인덱스"), index #7=27 ("인덱스")) -> (element #1=w688:string, element #2=w687:string, element #3=w686:string, element #4=w684:string, element #5=w683:string, element #6=w682:string, element #7=w685:string)  [unwired: 3 in]
      n211 = Index Array(array=w662) -> (element #1=w657:string, element #2=w661:string)  [unwired: 2 in]
      n212 = Build Array(w688, w687, w686, w684, w683, w685) -> (w681:string[])
      n213 = for {
        tunnel: w682 -> [w698]
        tunnel: w681 -> [w697] mode=indexing
        tunnel: w664 -> [w696]
        tunnel: [w695] -> w680 mode=indexing
        n214 = call "Unit Conversion.vi"("환산단위"=w696, "입력단위"=w698, "입력값"=w697) -> ("환산값 (string)"=w695:string)  [unwired: 3 in, 5 out]
      }
      n215 = Equal?(x=w661, y="담수") -> (x = y?=w659:bool)
      n216 = Index Array(array=w694, index (col)=2 ("비활성화된 인덱스 (열)")) -> (element=w692:string[])  [unwired: 1 in]
      n217 = Fract/Exp String To Number(string=w657) -> (number=w658:dbl)  [unwired: 3 in, 1 out]
      n218 = Index Array(array=w680) -> (element #1=w679:string, element #2=w678:string, element #3=w677:string, element #4=w676:string, element #5=w675:string, element #6=w674:string)  [unwired: 6 in]
      n219 = Replace Array Subset(array=w665, new element #1=w679, index #1=13 ("인덱스"), new element #2=w678, new element #3=w677, new element #4=w664, new element #5=w676, index #5=17 ("인덱스"), new element #6=w664, new element #7=w675, index #7=24 ("인덱스"), new element #8=w664, new element #9=w674, index #9=27 ("인덱스")) -> (w663:string[])  [unwired: 5 in]
      n220 = for {
        tunnel: w689 -> [w721] mode=indexing
        tunnel: [w720] -> w690 mode=indexing
        tunnel: w663 -> [w706]
        tunnel: [w719] -> w691 mode=indexing
        tunnel: w692 -> [w716] mode=indexing
        tunnel: w659 -> [w700]
        tunnel: w658 -> [w699]
        i -> [w715]
        n221 = Index Array(array=w721) -> (element #1=w717:string, element #2=w718:string)  [unwired: 2 in]
        n222 = Increment(x=w715) -> (x+1=w714:i32)
        n223 = Fract/Exp String To Number(string=w717) -> (number=w712:dbl)  [unwired: 3 in, 1 out]
        n224 = Number To Decimal String(number=w714) -> (decimal integer string=w713:string)  [unwired: 1 in]
        n225 = Index Array(array=w706, index #1=11 ("인덱스"), index #2=24 ("인덱스")) -> (element #1=w702:string, element #2=w707:string, element #3=w709:string, element #4=w708:string, element #5=w710:string)  [unwired: 3 in]
        n226 = Fract/Exp String To Number(string=w702) -> (number=w704:dbl)  [unwired: 3 in, 1 out]
        n227 = Equal To 0?(x=w712) -> (x = 0?=w705:bool)
        n228 = Less Or Equal?(x=w712, y=w704) -> (x <= y?=w711:bool)
        n229 = case shown="참" w711 {
          tunnel: [_ w764] -> w719
          tunnel: w713 -> [_ w751]
          tunnel: w706 -> [_ w754]
          tunnel: [_ w753] -> w720
          tunnel: w709 -> [_ w734]
          tunnel: w710 -> [_ w752]
          tunnel: w718 -> [_ w729]
          tunnel: w717 -> [_ w759]
          tunnel: w708 -> [_ w762]
          tunnel: w707 -> [_ _]
          tunnel: w716 -> [_ w735]
          tunnel: w705 -> [_ w750]
          tunnel: w700 -> [_ w732]
          tunnel: w699 -> [_ w725]
          frame False {
          }
          frame True {
            n230 = call "Number Format.vi"("기준단위"=w734, "입력단위"=w729, "입력값"=w735) -> ("정밀도(단위적용)"=w736:i32)  [unwired: 8 in]
            n231 = call "Number Format.vi"("기준단위"=w729, "입력단위"=w734, "입력값"=w735) -> ("정밀도(단위적용)"=w733:i32)  [unwired: 8 in]
            n232 = call "Unit Conversion.vi"("소수점 자리수"=w736, "환산단위"=w734, "입력단위"=w729, "입력값"=w759) -> ("환산단위"=w728:string, "환산값 (DBL)"=w763:dbl, "환산값 (string)"=w758:string)  [unwired: 2 in, 3 out]
            n233 = Fract/Exp String To Number(string=w762) -> (number=w761:dbl)  [unwired: 3 in, 1 out]
            n234 = Fract/Exp String To Number(string=w752) -> (number=w760:dbl)  [unwired: 3 in, 1 out]
            n235 = Multiply(x=w761, y=w763) -> (x*y=w765:dbl)
            n236 = Add(x=w765, y=w760) -> (x+y=w749:dbl)
            n237 = Select(t=0.0, s=w750, f=w749) -> (s? t:f=w747:dbl)
            n238 = Number To Fractional String(number=w747, precision (6)=w736) -> (F-format string=w730:string)  [unwired: 2 in]
            n239 = call "Unit Conversion.vi"("환산단위"=w729, "입력단위"=w728, "입력값"=w752) -> ("환산단위"=w741:string, "환산값 (string)"=w742:string)  [unwired: 3 in, 4 out]
            n240 = call "Unit Conversion.vi"("소수점 자리수"=w733, "환산단위"=w729, "입력단위"=w728, "입력값"=w758) -> ("환산값 (string)"=w757:string)  [unwired: 2 in, 5 out]
            n241 = call "Unit Conversion.vi"("소수점 자리수"=w733, "환산단위"=w729, "입력단위"=w728, "입력값"=w730) -> ("환산단위"=w755:string, "환산값 (DBL)"=w740:dbl, "환산값 (string)"=w756:string)  [unwired: 2 in, 3 out]
            n242 = call "Unit Conversion.vi"("환산단위"="Pa", "입력단위"=w728, "입력값"=w730) -> ("환산값 (DBL)"=w726:dbl)  [unwired: 3 in, 5 out]
            n243 = xnode ("수식")("p1_Pa"=w726, "t1_℃"=w725) -> ("결과"=w731:dbl)  [unwired: 1 in, 1 out]
            n244 = Replace Array Subset(array=w754, new element #1=w742, index #1=27 ("인덱스"), new element #2=w741, index #2=25 ("인덱스")) -> (w753:string[])
            n245 = Select(t=w731, s=w732, f=1.026 ("y")) -> (s? t:f=w722:dbl)
            n246 = Multiply(x=w722, y=9.80665 ("중력가속도")) -> (x*y=w745:dbl)
            n247 = Divide(x=w740, y=w745) -> (x/y=w724:dbl)
            n248 = Format Into String(format string="%.2f" ("포맷 문자열"), w724) -> (resulting string=w738:string)  [unwired: 2 in, 1 out]
            n249 = Build Array(w751, w757, w756, w755, w738, "m" ("원소")) -> (w764:string[])
          }
        }
      }
    }
  }
  "Data Out" <- w9
  "STD Data" <- w8
  "배열" <- w1
